vi "Get Channel Count.vi"(11 "DBL Buffer in":refnum<class "DBL Pointer.lvclass">) -> (2 "channel count":u64, 3 "DBL Buffer out":refnum<class "DBL Pointer.lvclass">)   [LabVIEW 2017, in "DSF Core.lvlib" / "DBL Pointer.lvclass"]
uses:
  DBL Pointer.lvclass
  DBL Pointer.lvclass/DBL Pointer.ctl
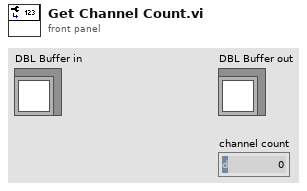
[diagram p1: front panel]
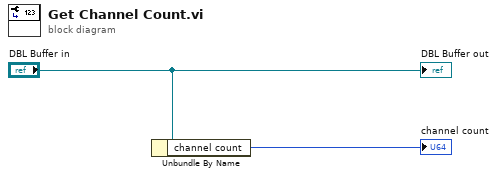
[diagram p0: block diagram]
diagram:
  n1 = Unbundle By Name("DBL Buffer in") -> ("channel count"=→"channel count":u64)
  "DBL Buffer out" <- "DBL Buffer in"
